vi "Gui_UpdateExperiment.vi"(5 "Laser 3.Energy":dbl, 7 "Laser 3.Wavelength":i16, 8 "error in (no error)":errorcluster, 10 "Variant Loops":variant, 11 "Variant Experiment":variant) -> (0 "error out":errorcluster caption="sortie d'erreur", 3 "Variant Output":variant)   [LabVIEW 2024]
doc: "This VI setup the parameters for the experiment.\n\n1. Init the controls with the previous values and update the list boxes and rings with external text files located in TECHNICAL\\RESOURCES directories : \"Users.txt\", \"Sources.txt\", etc.\n2. The controls are passed by a Variant in input.\n3. Wait for the user events, and update controls accordingly.\n4. When OK is pushed, return an updated Variant as output."
uses:
  controls/EXPERIMENT_Inputs.ctl
  controls/LASER_Inputs.ctl
  controls/LAMP_Inputs.ctl
  controls/GAS_Inputs.ctl
  controls/LOOPS_Inputs.ctl
  controls/OPO_Inputs.ctl
panel:
  in  "LOOPS Inputs":T1={"Number of Loops"=0, "Loop Current Value"=0, "OPO Inputs"={"OPO AutoAlignment ON"=FALSE, "OPO Start Value"=210.0, "OPO Stop Value"=270.0, "OPO Step"=30.0}} {"OPO Inputs"."OPO Step" min=0.5 max=60.0 format="%#.1f"; "OPO Inputs"."OPO Stop Value" min=210.0 max=270.0 format="%#.1f"; "OPO Inputs"."OPO Start Value" min=210.0 max=270.0 format="%#.1f"}
  in  "EXPERIMENT Inputs":T3={"Setup"="", "Date"="", "User Name"="", "Comment"="", "Experiment Procedures"=[], "Chemical Source"="", "Sample Components"=[], "Species"=[], "Laser 1"={"Used"=TRUE, "Name"="Spectroscopy", "Wavelength"=1000.0, "Energy"=25.0}, "Laser 2"={"Used"=TRUE, "Name"="Spectroscopy", "Wavelength"=1000.0, "Energy"=25.0}, "Laser 3"={"Used"=TRUE, "Name"="Spectroscopy", "Wavelength"=1000.0, "Energy"=25.0}, "Laser 4"={"Used"=TRUE, "Name"="Spectroscopy", "Wavelength"=1000.0, "Energy"=25.0}, "Laser 5"={"Used"=TRUE, "Name"="Spectroscopy", "Wavelength"=1000.0, "Energy"=25.0}, "Lamp 1"={"Used"=TRUE, "Name"="Spectroscopy", "Wavelength"=1000.0, "Attenuation"=25.0}, "Lamp 2"={"Used"=TRUE, "Name"="Spectroscopy", "Wavelength"=1000.0, "Attenuation"=25.0}, "Gas 1"={"Used"=TRUE, "Name"="Spectroscopy", "Pressure"=1000.0}, "Gas 2"={"Used"=TRUE, "Name"="Spectroscopy", "Pressure"=1000.0}, "Gas 3"={"Used"=TRUE, "Name"="Spectroscopy", "Pressure"=1000.0}, "Gas 4"={"Used"=TRUE, "Name"="Spectroscopy", "Pressure"=1000.0}, "Gas 5"={"Used"=TRUE, "Name"="Spectroscopy", "Pressure"=1000.0}}
  # "Lasers"
  # "nm"
  # "mJ"
  # "Lamps"
  # "nm"
  # "dB"
  # "Gas"
  # "bar"
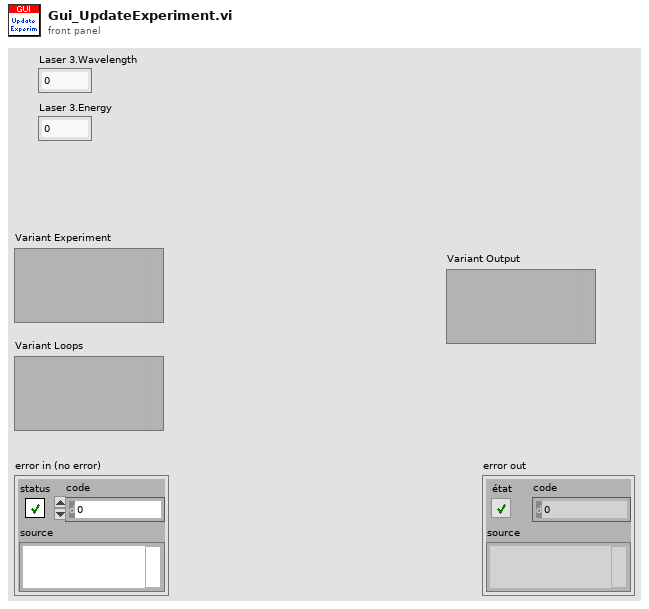
[diagram p1: front panel]
types:
  T1 = typedef "LOOPS_Inputs.ctl" = cluster{"Number of Loops":i16, "Loop Current Value":i16, "OPO Inputs":T2}
  T2 = typedef "OPO_Inputs.ctl" = cluster{"OPO AutoAlignment ON":bool, "OPO Start Value":dbl, "OPO Stop Value":dbl, "OPO Step":dbl}
  T3 = typedef "EXPERIMENT_Inputs.ctl" = cluster{"Setup":string, "Date":string, "User Name":string, "Comment":string, "Experiment Procedures":string[], "Chemical Source":string, "Sample Components":string[], "Species":string[], "Laser 1":T4, "Laser 2":T4, "Laser 3":T4, "Laser 4":T4, "Laser 5":T4, "Lamp 1":T5, "Lamp 2":T5, "Gas 1":T6, "Gas 2":T6, "Gas 3":T6, "Gas 4":T6, "Gas 5":T6}
  T4 = typedef "LASER_Inputs.ctl" = cluster{"Used":bool, "Name":string, "Wavelength":dbl, "Energy":dbl}
  T5 = typedef "LAMP_Inputs.ctl" = cluster{"Used":bool, "Name":string, "Wavelength":dbl, "Attenuation":dbl}
  T6 = typedef "GAS_Inputs.ctl" = cluster{"Used":bool, "Name":string, "Pressure":dbl}
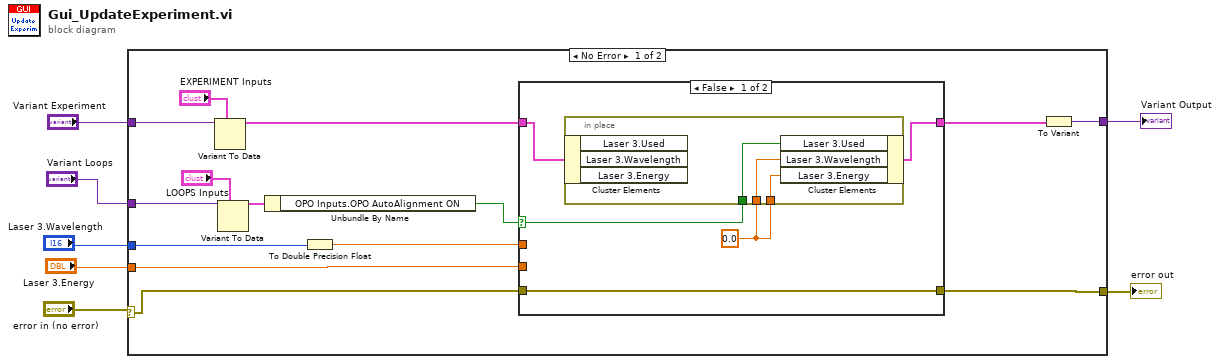
[diagram p0: block diagram]
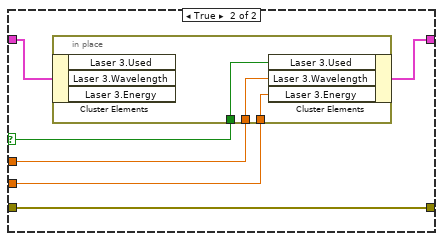
[diagram p2: hidden frame]
diagram:
  n1 = case shown="No Error" "error in (no error)" {
    selector: "error in (no error)" -> [w11 w39]
    tunnel: [w10 w39] -> w7
    tunnel: "Variant Experiment" -> [w20 w40]
    tunnel: [w21 w40] -> w5
    tunnel: "Variant Loops" -> [w18 _]
    tunnel: "Laser 3.Wavelength" -> [w9 _]
    tunnel: "Laser 3.Energy" -> [w12 _]
    frame No Error {
      n2 = Variant To Data(type="EXPERIMENT Inputs", Variant=w20) -> (data=w14:T3)  [unwired: 1 in, 1 out]
      n3 = Variant To Data(type="LOOPS Inputs", Variant=w18) -> (data=w16:T1)  [unwired: 1 in, 1 out]
      n4 = Unbundle By Name(w16) -> ("OPO Inputs.OPO AutoAlignment ON"=w15:bool)
      n5 = To Double Precision Float(number=w9) -> (double precision float=w8:dbl)
      n6 = case shown="False" w15 {
        selector: w15 -> [w23 w32]
        tunnel: w14 -> [w25 w35]
        tunnel: [w24 w34] -> w13
        tunnel: w8 -> [_ w33]
        tunnel: w12 -> [_ w31]
        tunnel: w11 -> [w26 w30]
        tunnel: [w26 w30] -> w10
        frame False {
          w22 = 0.0
          n7 = in-place {
            in-place-border: w23 -> [w29]
            in-place-border: w22 -> [w28]
            in-place-border: w22 -> [w27]
            n8 = in-place-cluster #1(w25) -> ()  [unwired: 3 out]
            n9 = in-place-cluster #1("Laser 3.Used"=w29, "Laser 3.Wavelength"=w28, "Laser 3.Energy"=w27) -> (w24:T3)
          }
        }
        frame True {
          n10 = in-place {
            in-place-border: w33 -> [w38]
            in-place-border: w32 -> [w37]
            in-place-border: w31 -> [w36]
            n11 = in-place-cluster #2(w35) -> ()  [unwired: 3 out]
            n12 = in-place-cluster #2("Laser 3.Used"=w37, "Laser 3.Wavelength"=w38, "Laser 3.Energy"=w36) -> (w34:T3)
          }
        }
      }
      n13 = To Variant(anything=w13) -> (Variant=w21:variant)
    }
    frame Error {
    }
  }
  "error out" <- w7
  "Variant Output" <- w5
